vi "Round Vertex.vi"(11 "Vertex in":T1={"Position"={"x"=0.0, "y"=0.0, "z"=0.0}, "UV"={"u"=0.0, "v"=0.0}, "Colour"=12517256} {"UV"."v" min=0 max=1 step=0.1; "UV"."u" min=0 max=1 step=0.1}) -> (3 "Vertex With Position Rounded":T1={"Position"={"x"=0.0, "y"=0.0, "z"=0.0}, "UV"={"u"=0.0, "v"=0.0}, "Colour"=12517256} {"UV"."v" min=0 max=1 step=0.1; "UV"."u" min=0 max=1 step=0.1})   [LabVIEW 2022 SP3, in "3D.lvlib"]
uses:
  3D.lvlib
  Vertex.ctl
  Vector 3D.ctl
  Raster/UV.ctl
  Raster/Raster.lvlib
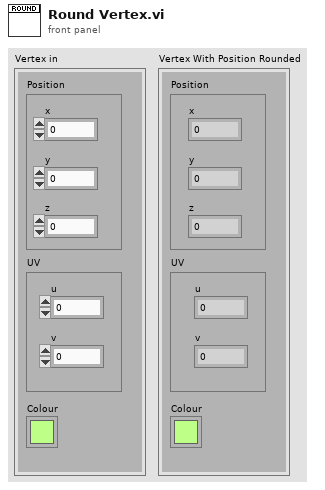
[diagram p1: front panel]
types:
  T1 = typedef "3D.lvlib/Vertex.ctl" = cluster{"Position":T2, "UV":T3, "Colour":u32}
  T2 = typedef "3D.lvlib/Vector 3D.ctl" = cluster{"x":sgl, "y":sgl, "z":sgl}
  T3 = typedef "Raster.lvlib/UV.ctl" = cluster{"u":sgl, "v":sgl}
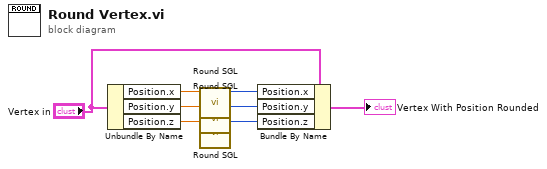
[diagram p0: block diagram]
diagram:
  n1 = Unbundle By Name("Vertex in") -> ("Position.x"=w6:sgl, "Position.y"=w4:sgl, "Position.z"=w2:sgl)
  n2 = call "Round SGL.vi"("SGL"=w6) -> ("I32"=w5:i32)  [unwired: 10 in]
  n3 = call "Round SGL.vi"("SGL"=w4) -> ("I32"=w3:i32)  [unwired: 10 in]
  n4 = call "Round SGL.vi"("SGL"=w2) -> ("I32"=w1:i32)  [unwired: 10 in]
  n5 = Bundle By Name(cluster="Vertex in", "Position.x"=w5, "Position.y"=w3, "Position.z"=w1) -> (→"Vertex With Position Rounded":T1)
